vi "IsInSafeLimitsXYZ.vi"(0 "XupLim":dbl=1199.0, 1 "ZupLim":dbl=99.0, 2 "Controller In":refnum<k24>, 5 "XlowLim":dbl, 7 "YupLim":dbl=1199.0, 9 "YlowLim":dbl, 11 "Error In":errorcluster, 12 "ZlowLim":dbl=-0.1) -> (3 "controller out":refnum<k24>, 4 "XYZinLimits":bool, 15 "Error Out":errorcluster)   [LabVIEW 2021]
uses:
  C:/Users/TTUHEP/Documents/LabVIEW/Other Models/2010/Bin/Aerotech.A3200.dll
  Other Models/2010/Bin/Aerotech.A3200.dll
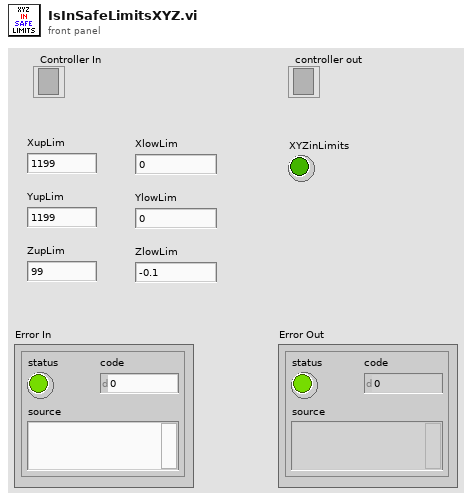
[diagram p1: front panel]
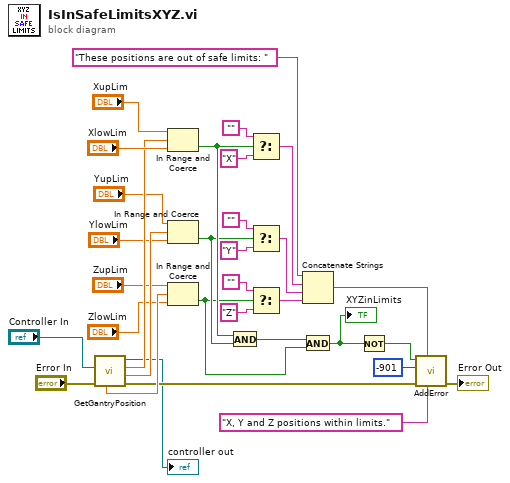
[diagram p0: block diagram]
diagram:
  n1 = call "GetGantryPosition.vi"("error in (no error)"="Error In", "Controller In"="Controller In") -> ("error out"=w8:errorcluster, "Position Y"=w30:dbl, "Position X"=w31:dbl, "controller out"=→"controller out":refnum<k24>, "Position Z"=w29:dbl)  [unwired: 3 in, 2 out]
  n2 = In Range and Coerce(upper limit="XupLim", x=w31, lower limit="XlowLim") -> (In Range?=w14:bool)  [unwired: 1 out]
  n3 = In Range and Coerce(upper limit="YupLim", x=w30, lower limit="YlowLim") -> (In Range?=w13:bool)  [unwired: 1 out]
  n4 = In Range and Coerce(upper limit="ZupLim", x=w29, lower limit="ZlowLim") -> (In Range?=w11:bool)  [unwired: 1 out]
  n5 = And(x=w14, y=w13) -> (x .and. y?=w12:bool)
  n6 = Select(t="", s=w14, f="X") -> (s? t:f=w21:string)
  n7 = Select(t="", s=w13, f="Y") -> (s? t:f=w16:string)
  n8 = Select(t="", s=w11, f="Z") -> (s? t:f=w15:string)
  n9 = Concatenate Strings("These positions are out of safe limits: " ("string"), w21, w16, w15) -> (w7:string)
  n10 = And(x=w12, y=w11) -> (x .and. y?=w4:bool)
  "XYZinLimits" <- w4
  n11 = Not(x=w4) -> (.not. x?=w10:bool)
  n12 = call "AddError.vi"("NoErrorMessage"="X, Y and Z positions within limits.", "ErrorMessage"=w7, "error in"=w8, "code"=-901, "Error?"=w10) -> ("Error out"=→"Error Out":errorcluster)  [unwired: 6 in]
